vi "Out_S6F12.vi"(8 "error in (no error)":errorcluster, 11 "S6 Message Class in":refnum<class "S6 Message Class.lvclass">) -> (0 "error out":errorcluster, 3 "S6 Message Class out":refnum<class "S6 Message Class.lvclass">)   [LabVIEW 2020, in "SECS Communication.lvlib" / "S6 Message Class.lvclass"]
uses:
  S6 Message Class.lvclass
  D:/Dropbox/SECS/SECS_GEM v1.0.6/Com/SECS Communication/SECS-II Class/SECS-II Class.lvclass
  SECS-II Class/Data Message_Binary.vi
  SECS-II Class/SECS-II Class.lvclass
  D:/Dropbox/SECS/SECS_GEM v1.0.6/Com/SECS Communication/S6 Message Class/S6 Message Class.lvclass
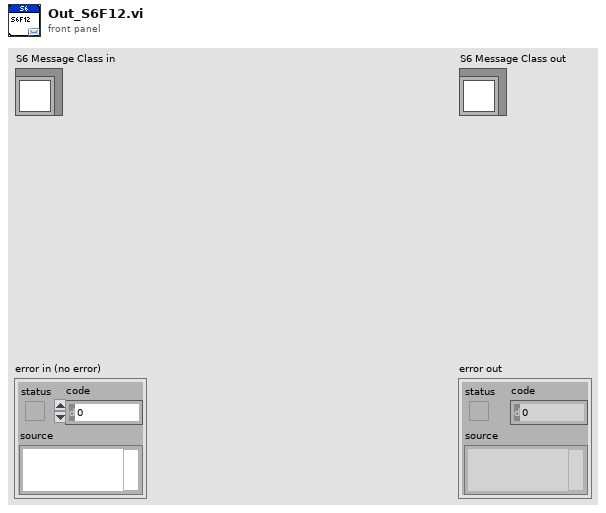
[diagram p1: front panel]
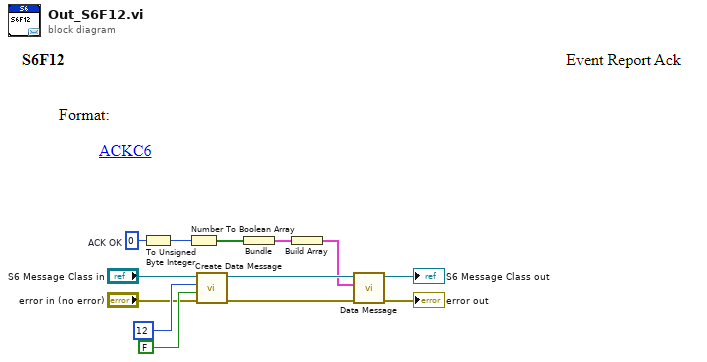
[diagram p0: block diagram]
diagram:
  w1 = u8 0  # ACK OK
  n1 = To Unsigned Byte Integer(number=w1) -> (unsigned 8bit integer=w9:u8)
  n2 = Number To Boolean Array(number=w9) -> (Boolean array=w8:bool[])
  n3 = call "Create Data Message.vi"("error in (no error)"="error in (no error)", "W-Bit"=FALSE, "Function"=u8 12, "SECS-II Class in"="S6 Message Class in") -> ("error out"=w10:errorcluster, "SECS-II Class out"=w11:refnum<class "S6 Message Class.lvclass">)  [unwired: 6 in]
  n4 = Bundle("Boolean array"=w8) -> (w7:cluster{"Boolean array":bool[]})  [unwired: 1 in]
  n5 = Build Array(w7) -> (w6:cluster{"Boolean array":bool[]}[])
  n6 = call-poly "Data Message.vi"("error in"=w10, "Data Cluster"=w6, "SECS-II Class in"=w11) -> ("error out"=→"error out":errorcluster, "SECS-II Class out"=→"S6 Message Class out":refnum<class "S6 Message Class.lvclass">)  [unwired: 7 in]
